vi "Read Multiline.vi"(8 "error in (no error)":errorcluster, 11 "Serializer.JSON in":refnum<class "Serializer.JSON.lvclass">) -> (0 "error out":errorcluster, 2 "Multiline":bool=TRUE, 3 "Serializer.JSON out":refnum<class "Serializer.JSON.lvclass">)   [LabVIEW 2019, in "OpenSerializer.JKI-JSON.lvlib" / "Serializer.JSON.lvclass"]
uses:
  Serializer.JSON.lvclass
  Serializer.JSON.lvclass/Serializer.JSON.ctl
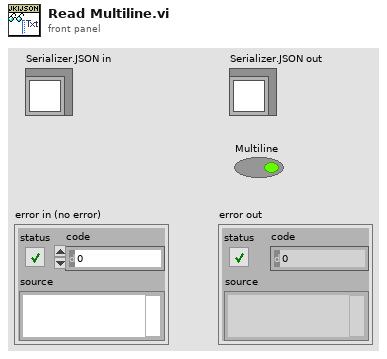
[diagram p1: front panel]
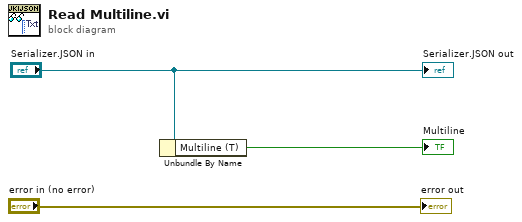
[diagram p0: block diagram]
diagram:
  n1 = Unbundle By Name("Serializer.JSON in") -> ("Multiline (T)"=→"Multiline":bool)
  "Serializer.JSON out" <- "Serializer.JSON in"
  "error out" <- "error in (no error)"
